vi "subBuildSpecifications.vi"(6 "ItemBuilt":refnum<user-event>, 7 "Preview?":bool, 8 "error in (no error)":errorcluster, 9 "Project refs":refnum<vi>[](array[refnum]), 10 "Local Host App Instance":refnum<vi>, 11 "Dependency order":T1[](array[typedef])) -> (0 "error out":errorcluster)   [LabVIEW 2020, in "SolutionBuilder.lvlib"]
uses:
  SolutionBuilder.lvlib
  FileInfo.ctl
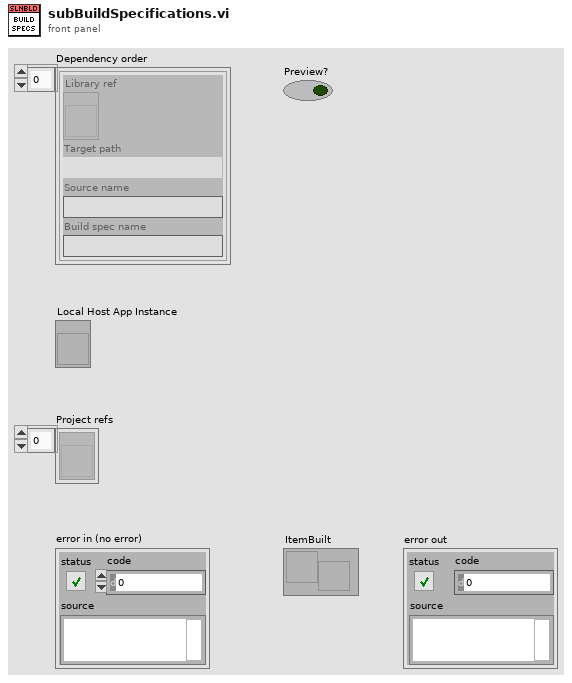
[diagram p1: front panel]
types:
  T1 = typedef "SolutionBuilder.lvlib/FileInfo.ctl" = cluster{"Library ref":refnum<vi>, "Target path":path, "Source name":string, "Build spec name":string}
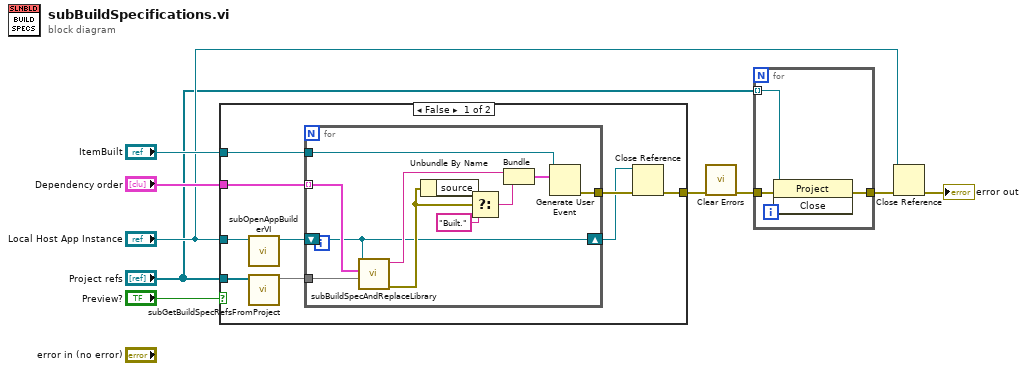
[diagram p0: block diagram]
diagram:
  n1 = case shown="False" "Preview?" {
    tunnel: "Dependency order" -> [w18 _]
    tunnel: "ItemBuilt" -> [w17 _]
    tunnel: "Local Host App Instance" -> [w11 _]
    tunnel: "Project refs" -> [w14 _]
    tunnel: [w10 _] -> w2
    frame False {
      n2 = call "subOpenAppBuilderVI.vi"("Application in"=w11) -> ("VI ref"=w16:refnum<vi>)  [unwired: 10 in]
      n3 = call "subGetBuildSpecRefsFromProject.vi"("Project refs"=w14) -> ("Build spec refs"=w15:map{string, refnum<vi>})  [unwired: 10 in]
      n4 = for {
        tunnel: w17 -> [w29]
        tunnel: w18 -> [w28] mode=indexing
        tunnel: [w24] -> w13
        tunnel: w15 -> [w21]
        shift-right: [w19] -> w12
        shift-left: w16 -> [w19]
        n5 = call "subBuildSpecAndReplaceLibrary.vi"("Build spec refs"=w21, "FileInfo"=w28, "VI in"=w19) -> ("error out"=w20:errorcluster, "Message"=w22:string)  [unwired: 7 in]
        n6 = Unbundle By Name(w20) -> ("source"=w26:string)
        n7 = Select(t=w26, s=w20, f="Built.") -> (s? t:f=w23:string)
        n8 = Bundle("Message"=w22, "f"=w23) -> (w27:cluster{"Message":string, "f":string})  [unwired: 1 in]
        n9 = Generate User Event(user event=w29, event data cluster=w27) -> (error out=w24:errorcluster)  [unwired: 2 in, 1 out]
      }
      n10 = Close Reference(reference=w12, error in (no error)=w13) -> (error out=w10:errorcluster)
    }
    frame True {
    }
  }
  n11 = call <vilib>:"Clear Errors.vi"("error in (no error)"=w2) -> ("error out"=w1:errorcluster)  [unwired: 5 in, 1 out]
  n12 = for {
    tunnel: "Project refs" -> [w31] mode=indexing
    tunnel: w1 -> [w32]
    tunnel: [w30] -> w4
    n13 = invoke class="Project" method="Close"(reference=w31, error in=w32) -> (error out=w30:errorcluster)  [unwired: 1 in, 2 out]
  }
  n14 = Close Reference(reference="Local Host App Instance", error in (no error)=w4) -> (error out=→"error out":errorcluster)
